vi "Clear Backlog Indicators.vi"(8 "error in (no error)":errorcluster, 11 "FP Controls in":refnum<class "FP Controls.lvclass">) -> (0 "error out":errorcluster, 3 "FP Controls out":refnum<class "FP Controls.lvclass">)   [LabVIEW 2018, in "Configuration Grandmaster.lvlib" / "FP Controls.lvclass"]
uses:
  FP Controls.lvclass
  Common/Controls/TE_Designator.ctl
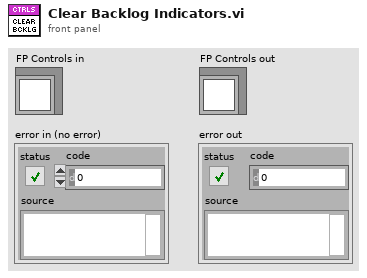
[diagram p1: front panel]
types:
  T1 = typedef "TE_Designator.ctl" = enum16{"High Speed", "Low Speed"}
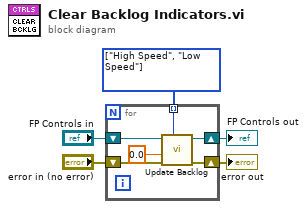
[diagram p0: block diagram]
diagram:
  w5 = T1[] [enum."High Speed", enum."Low Speed"] items=["High Speed", "Low Speed"]
  n1 = for {
    shift-right: [w7] -> w4
    shift-left: "FP Controls in" -> [w10]
    shift-right: [w8] -> w3
    shift-left: "error in (no error)" -> [w11]
    tunnel: w5 -> [w6] mode=indexing
    n2 = call "Update Backlog.vi"("TimingEngine"=w6, "error in (no error)"=w11, "Backlog"=0.0, "FP Controls in"=w10) -> ("error out"=w8:errorcluster, "FP Controls out"=w7:refnum<class "FP Controls.lvclass">)  [unwired: 6 in]
  }
  "FP Controls out" <- w4
  "error out" <- w3
